vi "Get FPGA Property Value.vi"(8 "error in (no error)":errorcluster, 10 "Property Name":string, 11 "FPGA Personality File Path":path) -> (0 "error out":errorcluster, 1 "Found?":bool, 2 "Property Value":string, 3 "Duplicated FPGA Personality File Path":path)   [LabVIEW 2021, in "Personality.lvlib"]
doc: "Gets the specified property value from the specified FPGA personality file."
uses:
  <vilib>/myRIO/Common/FPGA Personality Framework/Personality.lvlib
  <vilib>/xml/Load XML File.vi
  <vilib>/xml/Close Reference(Node).vi
  <vilib>/xml/NI_XML.lvlib
  <resource>/objmgr/DOMUserDefRef.rc
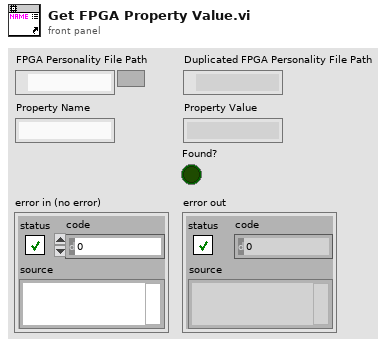
[diagram p1: front panel]
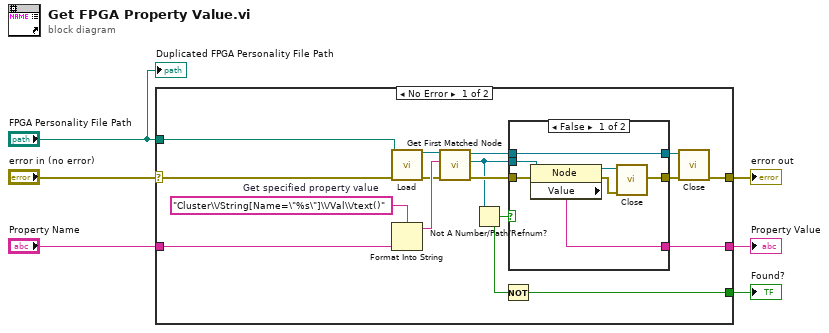
[diagram p0: block diagram]
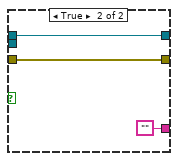
[diagram p2: hidden frame]
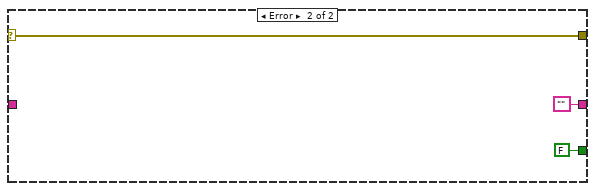
[diagram p3: hidden frame]
diagram:
  n1 = case shown="No Error" "error in (no error)" {
    selector: "error in (no error)" -> [w21 w35]
    tunnel: "Property Name" -> [w22 _]
    tunnel: [w20 w35] -> w4
    tunnel: "FPGA Personality File Path" -> [w19 _]
    tunnel: [w9 "" ("Value")] -> w3
    tunnel: [w7 FALSE] -> w2
    frame No Error {
      w17 = "Cluster\\/String[Name=\"%s\"]\\/Val\\/text()"  # Get specified property value
      n2 = call-poly <vilib>:"Load.vi"("path to XML document"=w19, "error in (no error)"=w21) -> ("DOM document out"=w18:refnum<k20>, "error out"=w15:errorcluster)  [unwired: 11 in, 1 out]
      n3 = Format Into String(format string=w17, w22) -> (resulting string=w16:string)  [unwired: 2 in, 1 out]
      n4 = call <vilib>:"Get First Matched Node.vi"("error in (no error)"=w15, "XPath expression"=w16, "node in"=w18) -> ("error out"=w14:errorcluster, "node result"=w12:refnum<k20>, "node out"=w13:refnum<k20>)  [unwired: 6 in]
      n5 = Not A Number/Path/Refnum?(number/path/refnum=w12) -> (NaN/Path/Refnum?=w8:bool)
      n6 = Not(x=w8) -> (.not. x?=w7:bool)
      n7 = case shown="False" w8 {
        tunnel: w14 -> [w28 w31]
        tunnel: w13 -> [w29 w32]
        tunnel: w12 -> [w26 _]
        tunnel: [w29 w32] -> w11
        tunnel: [w23 w31] -> w10
        tunnel: [w25 "" ("Value")] -> w9
        frame False {
          n8 = property class="Node"(reference=w26, error in=w28) -> (reference out=w24:refnum<k20>, error out=w27:errorcluster, "Value"=w25:string)
          n9 = call-poly <vilib>:"Close.vi"("error in (no error)"=w27, "node"=w24) -> ("error out"=w23:errorcluster)  [unwired: 7 in]
        }
        frame True {
        }
      }
      n10 = call-poly <vilib>:"Close.vi"("error in (no error)"=w10, "node"=w11) -> ("error out"=w20:errorcluster)  [unwired: 7 in]
    }
    frame Error {
    }
  }
  "Property Value" <- w3
  "error out" <- w4
  "Found?" <- w2
  "Duplicated FPGA Personality File Path" <- "FPGA Personality File Path"
